vi "fgt set manual.vi"(8 "error in (no error)":errorcluster, 10 "value":sgl=5.0, 11 "pressureIndex":u32) -> (0 "error out":errorcluster)   [LabVIEW 2020, in "fgt_SDK.lvlib"]
doc: "Manually activate internal electrovalve. This stops pressure regulation.\nThis feature is only available on MFCS and MFCS-EZ devices."
uses:
  fgt_SDK.lvlib
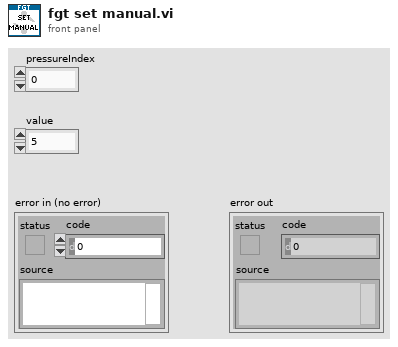
[diagram p1: front panel]
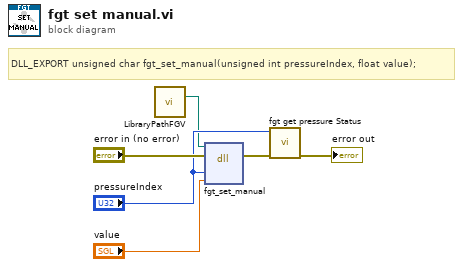
[diagram p0: block diagram]
diagram:
  # "DLL_EXPORT unsigned char fgt_set_manual(unsigned int pressureIndex, float value);"
  n1 = call "LibraryPathFGV.vi"() -> ("Path Out"=w1:path)  [unwired: 14 in, 1 out]
  n2 = dll-call lib="C:/Workspace/fgt-SDK/LabVIEW/dlls/fgt_SDK_*.*" fn="fgt_set_manual"(path in=w1, error in="error in (no error)", "pressureIndex"="pressureIndex", "value"="value") -> (error out=w4:errorcluster)  [unwired: 4 in, 1 out]
  n3 = call "fgt get pressure Status.vi"("error in (no error)"=w4, "pressureIndex"="pressureIndex") -> ("error out"=→"error out":errorcluster)  [unwired: 9 in]
